vi "Pilot Insertion.vi"(1 "Samples/Symbol":i32 min=2 step=2, 2 "Y(f) in":cdb[](array[numeric])) -> (0 "Y(f) out":cdb[](array[numeric]))   [LabVIEW 2018]
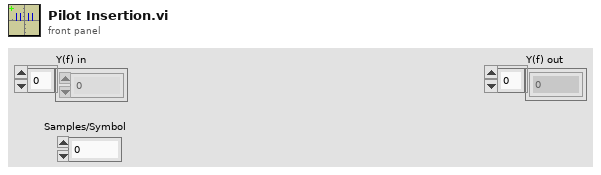
[diagram p1: front panel]
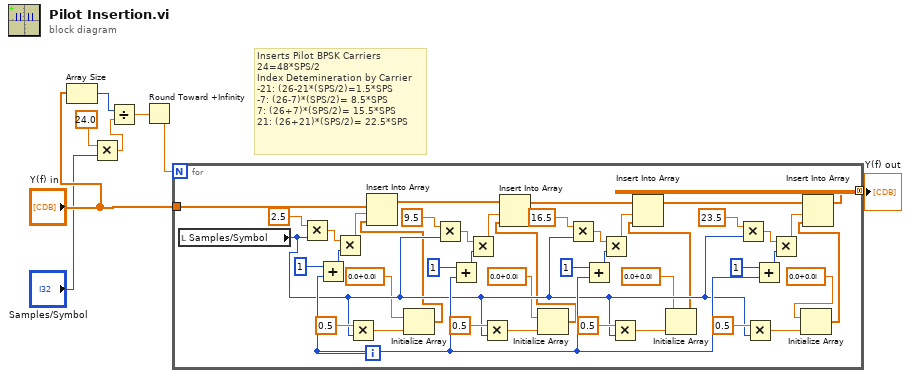
[diagram p0: block diagram]
diagram:
  # "Inserts Pilot BPSK Carriers\n24=48*SPS/2\nIndex Detemineration by Carrier\n-21: (26-21*(SPS/2)=1.5*SPS\n-7: (26-7)*(SPS/2)= 8.5*SPS\n7: (26+7)*(SPS/2)= 15.5*SPS\n21: (26+21)*(SPS/2)= 22.5*SPS"
  n1 = Array Size(array="Y(f) in") -> (size(s)=w7:i32)
  n2 = Multiply(x=24.0 ("y"), y="Samples/Symbol") -> (x*y=w1:dbl)
  n3 = Divide(x=w7, y=w1) -> (x/y=w8:dbl)
  n4 = Round Toward +Infinity(x=w8) -> (ceil(x): smallest int >= x=w6:dbl)
  n5 = for {
    N: w6 -> [_]
    tunnel: "Y(f) in" -> [w51]
    tunnel: [w30] -> w4 mode=concatenating
    i -> [w26]
    n6 = local read "Samples/Symbol"() -> (w17:i32)
    n7 = Multiply(x=2.5 ("index"), y=w17) -> (x*y=w47:dbl)
    n8 = Add(x=1, y=w26) -> (x+y=w46:i32)
    n9 = Multiply(x=w47, y=w46) -> (x*y=w48:dbl)
    n10 = Multiply(x=0.5, y=w17) -> (x*y=w24:dbl)
    n11 = Initialize Array(cdb 0.0+0.0i ("new element/subarray"), w24) -> (w9:cdb[])
    n12 = Insert Into Array(array=w51, index=w48, new element=w9) -> (w29:cdb[])
    n13 = Multiply(x=9.5 ("index"), y=w17) -> (x*y=w41:dbl)
    n14 = Add(x=1, y=w26) -> (x+y=w45:i32)
    n15 = Multiply(x=w41, y=w45) -> (x*y=w44:dbl)
    n16 = Multiply(x=0.5, y=w17) -> (x*y=w23:dbl)
    n17 = Initialize Array(cdb 0.0+0.0i ("new element/subarray"), w23) -> (w10:cdb[])
    n18 = Insert Into Array(array=w29, index=w44, new element=w10) -> (w28:cdb[])
    n19 = Multiply(x=16.5 ("index"), y=w17) -> (x*y=w40:dbl)
    n20 = Add(x=1, y=w26) -> (x+y=w36:i32)
    n21 = Multiply(x=w40, y=w36) -> (x*y=w37:dbl)
    n22 = Multiply(x=0.5, y=w17) -> (x*y=w20:dbl)
    n23 = Initialize Array(cdb 0.0+0.0i ("new element/subarray"), w20) -> (w11:cdb[])
    n24 = Insert Into Array(array=w28, index=w37, new element=w11) -> (w27:cdb[])
    n25 = Multiply(x=23.5 ("index"), y=w17) -> (x*y=w31:dbl)
    n26 = Multiply(x=0.5, y=w17) -> (x*y=w19:dbl)
    n27 = Add(x=1, y=w26) -> (x+y=w35:i32)
    n28 = Multiply(x=w31, y=w35) -> (x*y=w34:dbl)
    n29 = Initialize Array(cdb 0.0+0.0i ("new element/subarray"), w19) -> (w12:cdb[])
    n30 = Insert Into Array(array=w27, index=w34, new element=w12) -> (w30:cdb[])
  }
  "Y(f) out" <- w4
